vi "Digital Write by Name.vi"(8 "error in (no error)":errorcluster, 9 "Digital Data":bool, 10 "Channel Name":string, 11 "Digital Writer in":refnum<class "Digital Writer.lvclass">) -> (0 "error out":errorcluster, 3 "Digital Writer out":refnum<class "Digital Writer.lvclass">)   [LabVIEW 2024, in "DAQmx Actor.lvlib" / "Digital Writer.lvclass"]
uses:
  Digital Writer.lvclass
  Digital Writer.lvclass/Digital Writer.ctl
  <resource>/objmgr/daqmx.rc
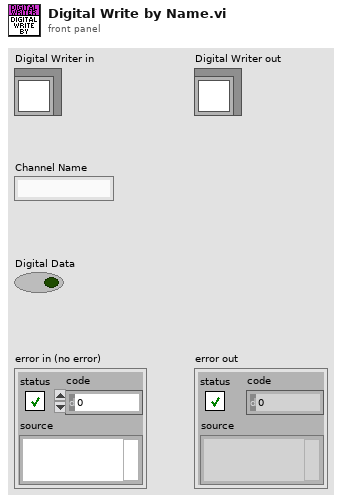
[diagram p1: front panel]
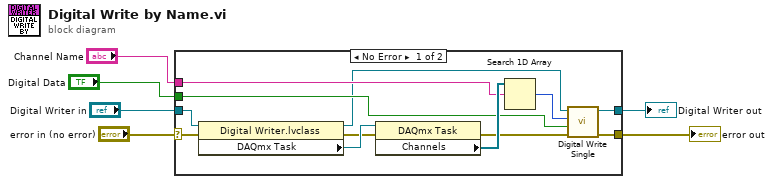
[diagram p0: block diagram]
diagram:
  n1 = case shown="No Error" "error in (no error)" {
    selector: "error in (no error)" -> [w10 w20]
    tunnel: [w9 w20] -> w5
    tunnel: [w7 w19] -> w3
    tunnel: "Digital Writer in" -> [w18 w19]
    tunnel: "Channel Name" -> [w15 _]
    tunnel: "Digital Data" -> [w13 _]
    frame No Error {
      n2 = property class="Digital Writer.lvclass"(reference=w18, error in=w10) -> (reference out=w8:refnum<class "Digital Writer.lvclass">, error out=w11:errorcluster, "DAQmx Task"=w17:refnum<k21>)
      n3 = property class="DAQmx Task"(reference=w17, error in=w11) -> (error out=w12:errorcluster, "Channels"=w16:refnum<k21>[])  [unwired: 1 out]
      n4 = Search 1D Array(1D array=w16, element=w15) -> (index of element=w14:i32)  [unwired: 1 in]
      n5 = call-dynamic "Digital Write Single.vi"("error in (no error)"=w12, "Digital Data"=w13, "Channel Index"=w14, "Digital Writer in"=w8) -> ("error out"=w9:errorcluster, "Digital Writer out"=w7:refnum<class "Digital Writer.lvclass">)  [unwired: 6 in]
    }
    frame Error {
    }
  }
  "error out" <- w5
  "Digital Writer out" <- w3
